vi "Finish Time Series.vi"(9 "Logging Cluster":T1={"Image Data Array"=[], "Buffer Number"=0, "Timestamp (um)"=0, "Exp params"={"Experiment Type"="Dynamic Time Series", "Experiment Name"="Experiment_1", "ExpPath"=path "D:/Data", "Save As"="TIFF", "TSFrames"=1000, "TSfps"=1.0, "Streaming"=FALSE, "tdms ref"=refnum, "frame #"=0, "Full Path"=path "", "PeakOnQueue"=FALSE}} {"Exp params"."TSFrames" min=1 step=1; "Exp params"."TSfps" min=0.001 max=90.0 step=0.001 format="%_4g"}, 10 "Session In":T3, 11 "Queue in":refnum<queue>) -> ()   [LabVIEW 2020]
uses:
  _controls/Logging Cluster.ctl
  _controls/Exp Params.ctl
  <vilib>/userDefined/High Color/IMAQdx.ctl
  <vilib>/vision/driver/IMAQdx.llb/IMAQdx Buffer Number Mode.ctl
  <vilib>/vision/driver/NI_Vision_Acquisition_Software.lvlib
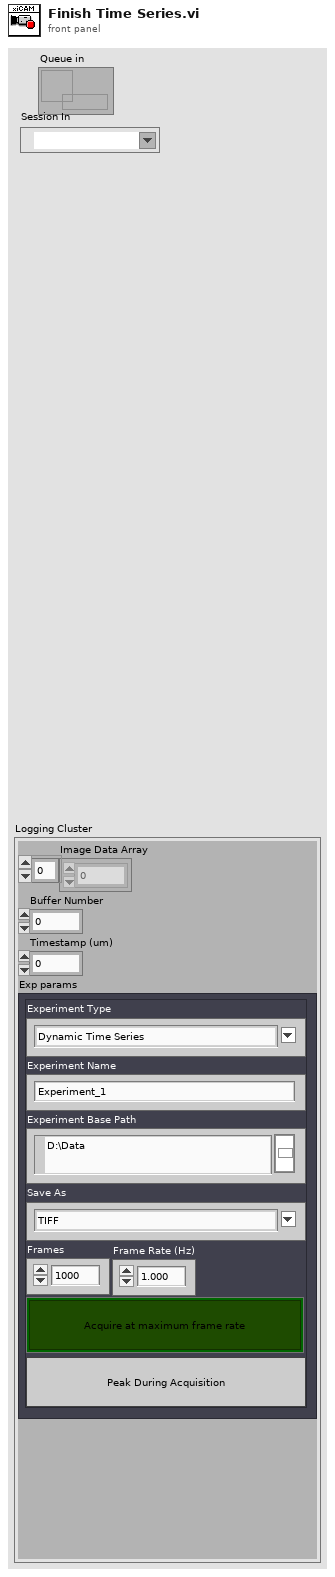
[diagram p1: front panel]
types:
  T1 = typedef "Logging Cluster.ctl" = cluster{"Image Data Array":u8[], "Buffer Number":i32, "Timestamp (um)":u64, "Exp params":T2}
  T2 = typedef "Exp Params.ctl" = cluster{"Experiment Type":string, "Experiment Name":string, "ExpPath":path, "Save As":string, "TSFrames":i32, "TSfps":dbl, "Streaming":bool, "tdms ref":refnum<k34>, "frame #":i64, "Full Path":path, "PeakOnQueue":bool}
  T3 = typedef "IMAQdx.ctl" = refnum<k21>
  T4 = typedef "NI_Vision_Acquisition_Software.lvlib/IMAQdx Buffer Number Mode.ctl" = enum32{"Next", "Last", "Buffer Number", "Every", "Last New"}
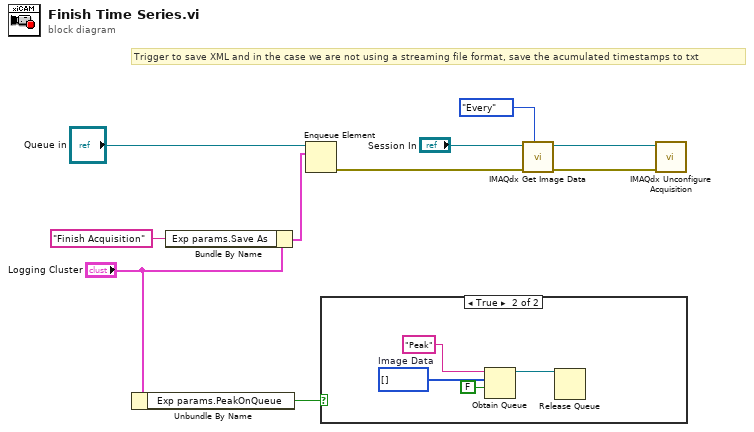
[diagram p0: block diagram]
diagram:
  # "Trigger to save XML and in the case we are not using a streaming file format, save the acumulated timestamps to txt"
  n1 = Unbundle By Name("Logging Cluster") -> ("Exp params.PeakOnQueue"=w2:bool)
  n2 = Bundle By Name(cluster="Logging Cluster", "Exp params.Save As"="Finish Acquisition") -> (w10:T1)
  n3 = Enqueue Element(queue="Queue in", element=w10) -> (error out=w5:errorcluster)  [unwired: 2 in, 2 out]
  n4 = case shown="True" w2 {
    frame False {
    }
    frame True {
      w14 = u8[] []  # Image Data
      n5 = Obtain Queue(name (unnamed)="Peak", element data type=w14, create if not found? (T)=FALSE) -> (queue out=w11:refnum<queue>)  [unwired: 2 in, 2 out]
      n6 = Release Queue(queue=w11) -> ()  [unwired: 2 in, 3 out]
    }
  }
  n7 = call <vilib>:"IMAQdx Get Image Data.vi"("Buffer Number Mode (Next)"=IMAQdx_Buffer_Number_Mode."Every", "error in"=w5, "Session In"="Session In") -> ("error out"=w3:errorcluster, "Session Out"=w4:T3)  [unwired: 5 in, 2 out]
  n8 = call <vilib>:"IMAQdx Unconfigure Acquisition.vi"("error in"=w3, "Session In"=w4) -> ()  [unwired: 8 in, 2 out]
